vi "ATF Storage-Enqueue Message_R.vi"(6 "Priority Message? (F)":bool, 8 "error in (no error)":errorcluster, 9 "Message Data":variant, 10 "Message":string, 11 "Message Queue":refnum<queue>) -> (0 "error out":errorcluster, 3 "dup Message Queue":refnum<queue>)   [LabVIEW 2022 SP3]
uses:
  RT Controls/ATF Storage-Message Cluster_R.ctl
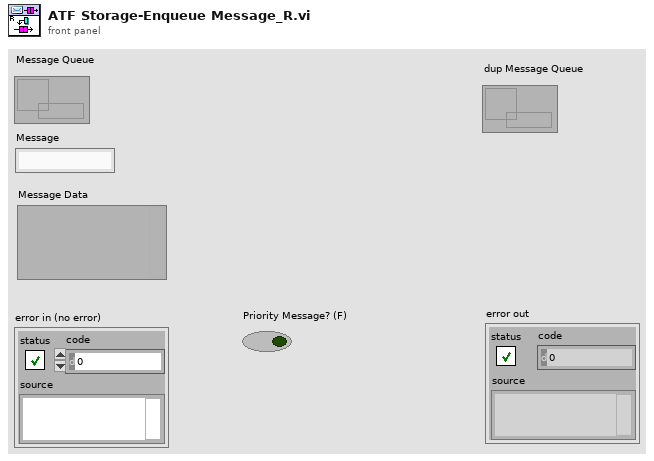
[diagram p1: front panel]
types:
  T1 = typedef "ATF Storage-Message Cluster_R.ctl" = cluster{"Message":string, "Message Data":variant}
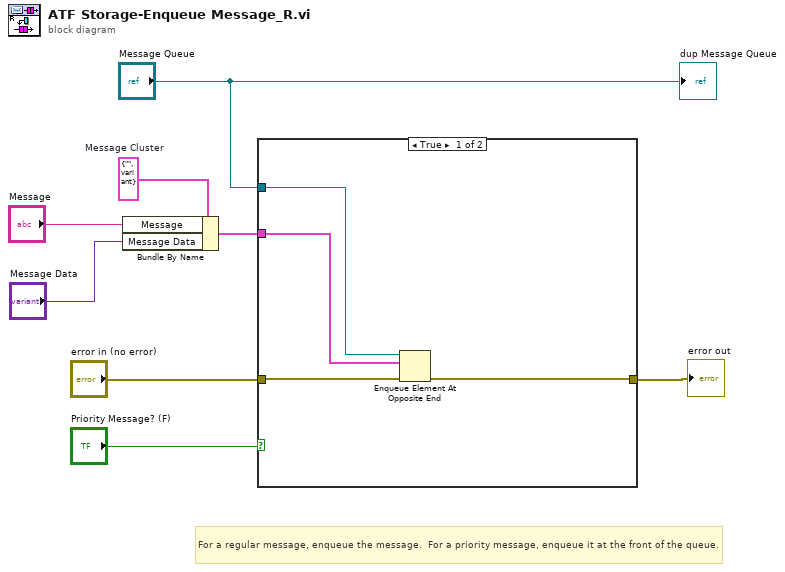
[diagram p0: block diagram]
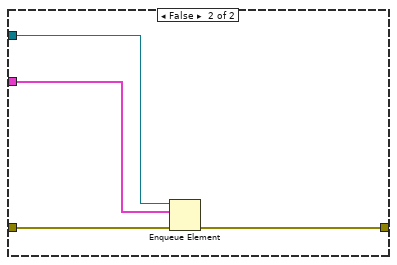
[diagram p2: hidden frame]
diagram:
  w5 = T1 {"Message"="", "Message Data"=variant}  # Message Cluster
  # "For a regular message, enqueue the message.  For a priority message, enqueue it at the front of the queue."
  n1 = Bundle By Name(cluster=w5, "Message"="Message", "Message Data"="Message Data") -> (w3:T1)
  n2 = case shown="True" "Priority Message? (F)" {
    tunnel: "error in (no error)" -> [w12 w16]
    tunnel: [w11 w15] -> w6
    tunnel: w3 -> [w9 w14]
    tunnel: "Message Queue" -> [w10 w13]
    frame True {
      n3 = Enqueue Element At Opposite End(queue=w10, element=w9, error in (no error)=w12) -> (error out=w11:errorcluster)  [unwired: 1 in, 2 out]
    }
    frame False {
      n4 = Enqueue Element(queue=w13, element=w14, error in (no error)=w16) -> (error out=w15:errorcluster)  [unwired: 1 in, 2 out]
    }
  }
  "error out" <- w6
  "dup Message Queue" <- "Message Queue"
